vi "Brass Logging.vi"(0 "GEA2 Reference In":refnum<k24>, 5 "Standalone?":bool, 7 "Board Index":i32, 11 "Error In":errorcluster) -> (4 "GEA2 Reference Out":refnum<k24>, 6 "Brass Logging":T1={"Basket speed"=0, "Shaft Speed"=0, "Folding"=0, "Jerk"=0, "Jerk Delta"=0, "State"="Unknown", "Counter"=0, "Motor Current"=0.0}, 15 "Error Out":errorcluster)   [LabVIEW 2016, in "TLMB.lvlib"]
uses:
  Projects/TLMB.lvlib
  Q:/Common/DLLs/GEA3/GeaCommunication.dll
  Common/DLLs/GEA3/GeaCommunication.dll
  Common/LabVIEW GEA2 Toolkit/LabVIEW_GEA2_Toolkit.lvlibp/type defs/Data Out.ctl
  type defs/Brass_Logging.ctl
  Common/LabVIEW GEA2 Toolkit/LabVIEW_GEA2_Toolkit.lvlibp/type defs/Source_Destination.ctl
  Common/LabVIEW GEA2 Toolkit/LabVIEW_GEA2_Toolkit.lvlibp
panel:
  in  "Brass Logging":T1={"Basket speed"=0, "Shaft Speed"=0, "Folding"=0, "Jerk"=0, "Jerk Delta"=0, "State"="Accel", "Counter"=0, "Motor Current"=0.0}
  out "Coverted Data Out":T2 {"CRC" format="%04x"; "Length" format="%02x"; "Command" format="%02x"; "Destination" format="%02x"; "Source" format="%02x"}
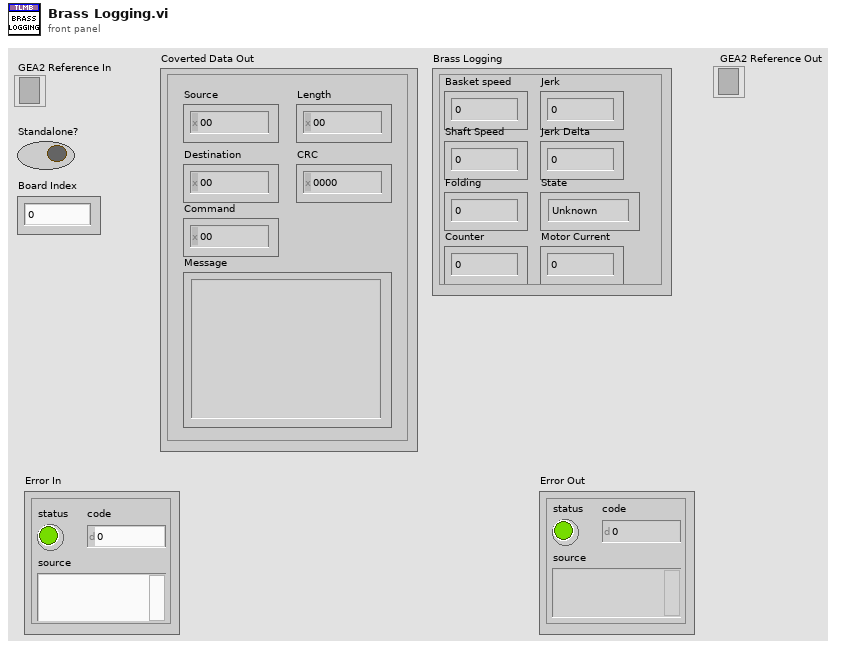
[diagram p1: front panel]
types:
  T1 = typedef "TLMB.lvlib/Brass_Logging.ctl" = cluster{"Basket speed":u16, "Shaft Speed":u16, "Folding":i32, "Jerk":i32, "Jerk Delta":u32, "State":string, "Counter":u8, "Motor Current":dbl}
  T2 = typedef "LabVIEW_GEA2_Toolkit.lvlibp/Data Out.ctl" = cluster{"Source":u8, "Destination":u8, "Command":u8, "Length":u8, "CRC":u16, "Message":string}
  T3 = typedef "LabVIEW_GEA2_Toolkit.lvlibp/Source_Destination.ctl" = cluster{"Source":u8, "Destination":u8}
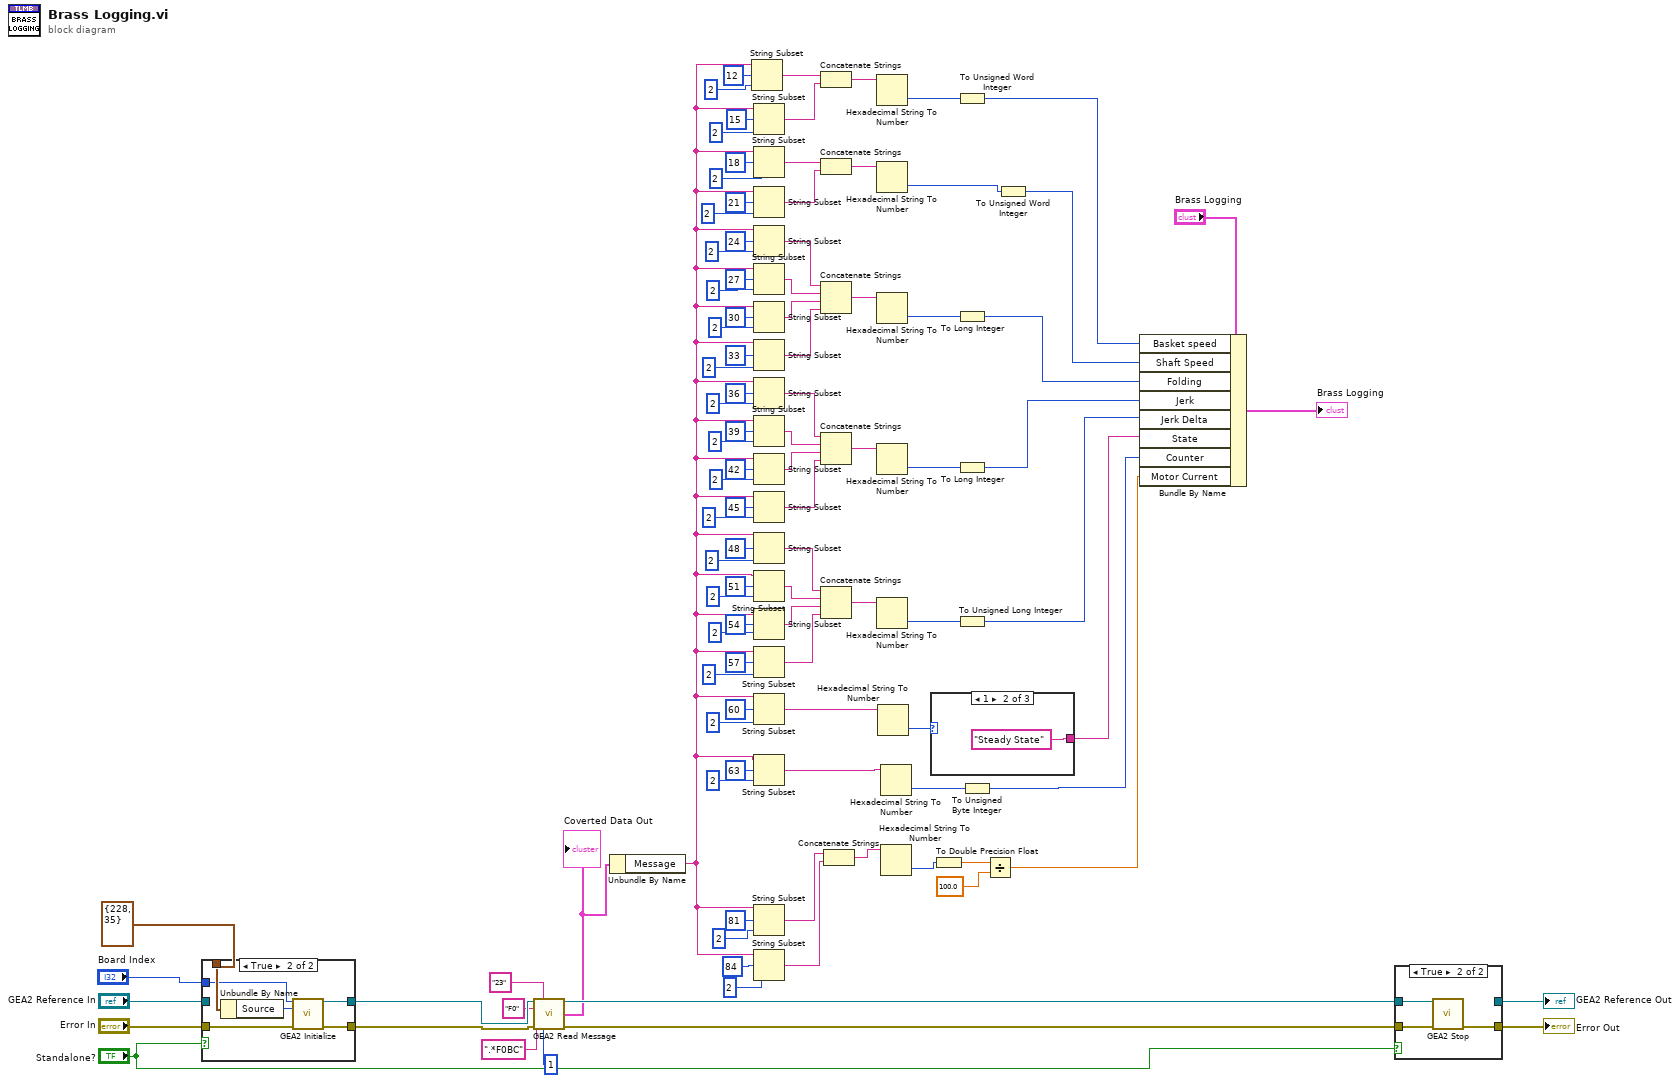
[diagram p0: block diagram]
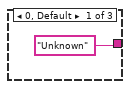
[diagram p2: hidden frame]
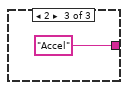
[diagram p3: hidden frame]
diagram:
  n1 = case shown="True" "Standalone?" {
    tunnel: "Error In" -> [w104 w111]
    tunnel: [w104 w110] -> w100
    tunnel: "GEA2 Reference In" -> [w105 _]
    tunnel: [w105 w109] -> w101
    tunnel: T3 {"Source"=228, "Destination"=35} ("GEA Inputs") -> [_ w107]
    tunnel: "Board Index" -> [_ w106]
    frame False {
    }
    frame True {
      n2 = Unbundle By Name(w107) -> ("Source"=w108:u8)
      n3 = call "GEA2 Initialize.vi"("Board Index"=w106, "Source Address"=w108, "error in"=w111) -> ("GEA2 Reference Out"=w109:refnum<k24>, "error out"=w110:errorcluster)  [unwired: 10 in, 1 out]
    }
  }
  n4 = call "GEA2 Read Message.vi"("GEA2 Reference In"=w101, "Expected Source"="23", "Expected Command"="F0", "Expected Data"=".*F0BC", "Error In"=w100, "# of Tries"=u8 1) -> ("GEA2 Reference Out"=w98:refnum<k24>, "Coverted Data Out"=w90:T2, "Error Out"=w97:errorcluster)  [unwired: 6 in, 1 out]
  "Coverted Data Out" <- w90
  n5 = Unbundle By Name(w90) -> ("Message"=w11:string)
  n6 = String Subset(string=w11, offset (0)=12, length (rest)=2 ("length (rest)")) -> (substring=w83:string)
  n7 = String Subset(string=w11, offset (0)=15, length (rest)=2 ("length (rest)")) -> (substring=w82:string)
  n8 = String Subset(string=w11, offset (0)=18, length (rest)=2 ("length (rest)")) -> (substring=w77:string)
  n9 = String Subset(string=w11, offset (0)=21, length (rest)=2 ("length (rest)")) -> (substring=w76:string)
  n10 = String Subset(string=w11, offset (0)=24, length (rest)=2 ("length (rest)")) -> (substring=w67:string)
  n11 = String Subset(string=w11, offset (0)=27, length (rest)=2 ("length (rest)")) -> (substring=w66:string)
  n12 = String Subset(string=w11, offset (0)=30, length (rest)=2 ("length (rest)")) -> (substring=w65:string)
  n13 = String Subset(string=w11, offset (0)=33, length (rest)=2 ("length (rest)")) -> (substring=w64:string)
  n14 = String Subset(string=w11, offset (0)=36, length (rest)=2 ("length (rest)")) -> (substring=w55:string)
  n15 = String Subset(string=w11, offset (0)=39, length (rest)=2 ("length (rest)")) -> (substring=w54:string)
  n16 = String Subset(string=w11, offset (0)=42, length (rest)=2 ("length (rest)")) -> (substring=w53:string)
  n17 = String Subset(string=w11, offset (0)=45, length (rest)=2 ("length (rest)")) -> (substring=w52:string)
  n18 = String Subset(string=w11, offset (0)=48, length (rest)=2 ("length (rest)")) -> (substring=w43:string)
  n19 = String Subset(string=w11, offset (0)=51, length (rest)=2 ("length (rest)")) -> (substring=w42:string)
  n20 = String Subset(string=w11, offset (0)=54, length (rest)=2 ("length (rest)")) -> (substring=w41:string)
  n21 = String Subset(string=w11, offset (0)=57, length (rest)=2 ("length (rest)")) -> (substring=w40:string)
  n22 = String Subset(string=w11, offset (0)=60, length (rest)=2 ("length (rest)")) -> (substring=w30:string)
  n23 = String Subset(string=w11, offset (0)=63, length (rest)=2 ("length (rest)")) -> (substring=w28:string)
  n24 = String Subset(string=w11, offset (0)=81, length (rest)=2 ("length (rest)")) -> (substring=w10:string)
  n25 = String Subset(string=w11, offset (0)=84, length (rest)=2 ("length (rest)")) -> (substring=w9:string)
  n26 = Concatenate Strings(w83, w82) -> (w35:string)
  n27 = Concatenate Strings(w77, w76) -> (w34:string)
  n28 = Concatenate Strings(w67, w66, w65, w64) -> (w33:string)
  n29 = Concatenate Strings(w55, w54, w53, w52) -> (w32:string)
  n30 = Concatenate Strings(w43, w42, w41, w40) -> (w31:string)
  n31 = Concatenate Strings(w10, w9) -> (w12:string)
  n32 = Hexadecimal String To Number(string=w35) -> (number=w27:u32)  [unwired: 2 in, 1 out]
  n33 = Hexadecimal String To Number(string=w34) -> (number=w13:u32)  [unwired: 2 in, 1 out]
  n34 = Hexadecimal String To Number(string=w33) -> (number=w26:u32)  [unwired: 2 in, 1 out]
  n35 = Hexadecimal String To Number(string=w32) -> (number=w25:u32)  [unwired: 2 in, 1 out]
  n36 = Hexadecimal String To Number(string=w31) -> (number=w24:u32)  [unwired: 2 in, 1 out]
  n37 = Hexadecimal String To Number(string=w30) -> (number=w29:u32)  [unwired: 2 in, 1 out]
  n38 = Hexadecimal String To Number(string=w28) -> (number=w23:u32)  [unwired: 2 in, 1 out]
  n39 = Hexadecimal String To Number(string=w12) -> (number=w2:u32)  [unwired: 2 in, 1 out]
  n40 = case shown="1" w29 {
    tunnel: ["Unknown" "Steady State" "Accel"] -> w16
    frame 0, Default {
    }
    frame 1 {
    }
    frame 2 {
    }
  }
  n41 = To Double Precision Float(number=w2) -> (double precision float=w1:dbl)
  n42 = To Unsigned Word Integer(number=w27) -> (unsigned 16bit integer=w21:u16)
  n43 = To Long Integer(number=w26) -> (32bit integer=w19:i32)
  n44 = To Long Integer(number=w25) -> (32bit integer=w18:i32)
  n45 = To Unsigned Long Integer(number=w24) -> (unsigned 32bit integer=w17:u32)
  n46 = To Unsigned Byte Integer(number=w23) -> (unsigned 8bit integer=w15:u8)
  n47 = Divide(x=w1, y=100.0) -> (x/y=w3:dbl)
  n48 = To Unsigned Word Integer(number=w13) -> (unsigned 16bit integer=w20:u16)
  n49 = Bundle By Name(cluster="Brass Logging", "Basket speed"=w21, "Shaft Speed"=w20, "Folding"=w19, "Jerk"=w18, "Jerk Delta"=w17, "State"=w16, "Counter"=w15, "Motor Current"=w3) -> (→"Brass Logging":T1)
  n50 = case shown="True" "Standalone?" {
    tunnel: [w116 w119] -> w95
    tunnel: w97 -> [w116 w118]
    tunnel: w98 -> [w115 w117]
    tunnel: [w115 _] -> w96
    frame False {
    }
    frame True {
      n51 = call "GEA2 Stop.vi"("GEA2 Reference In"=w117, "Error In"=w118) -> ("Error Out"=w119:errorcluster)  [unwired: 13 in]
    }
  }
  "GEA2 Reference Out" <- w96
  "Error Out" <- w95
